vi "MOKE-4-27-22.vi"() -> ()   [LabVIEW 2021]
uses:
  <vilib>/Analysis/NI_AALBase.lvlib
  <vilib>/Analysis/baseanly.llb/Mean (DBL).vi
  <vilib>/Analysis/Matrix/Datatypes/RealMatrix.ctl
  <vilib>/Analysis/Matrix/NI_Matrix.lvlib
panel:
  out "avg":dbl
  out "y_indicator":dbl
  out "col_arr":dbl[][](array[numeric])
  in  "blank":dbl[](array[numeric])
  out "y_mat":T1
  in  "stop":bool
  in  "Total Loops":dbl
  out "Current Loop":i32
  in  "Time / Step":i64
  in  "Number of Samples":i32=100
  out "Graph For Photodiode":cluster{"Y":dbl[], "Y":dbl[]}[](graph)
  out "Photodiode Level":dbl
  out "Current Voltage":dbl
  in  "Scans From 0 to Max Voltage":i32
  in  "Voltage":dbl
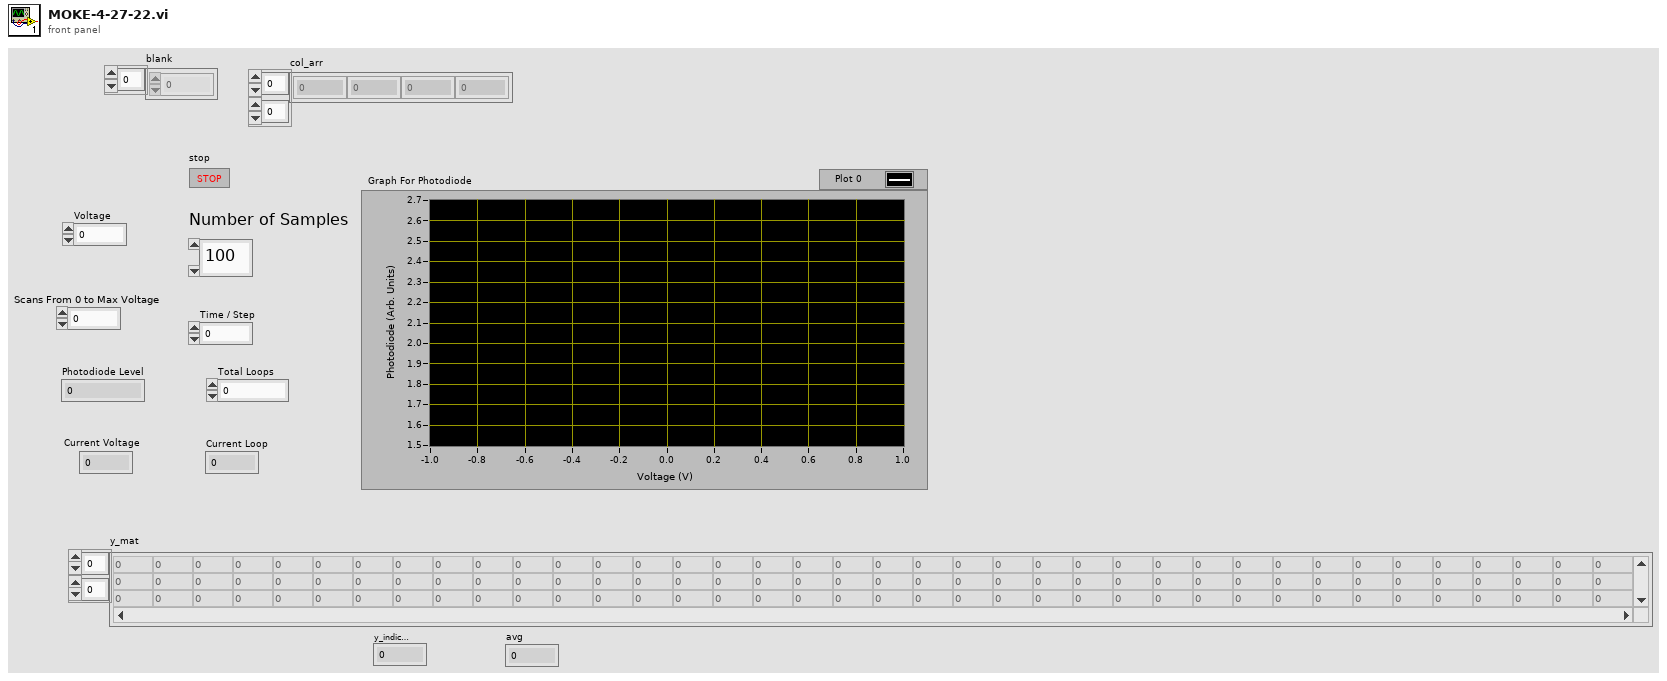
[diagram p1: front panel]
types:
  T1 = typedef "NI_Matrix.lvlib/RealMatrix.ctl" = dbl[][]
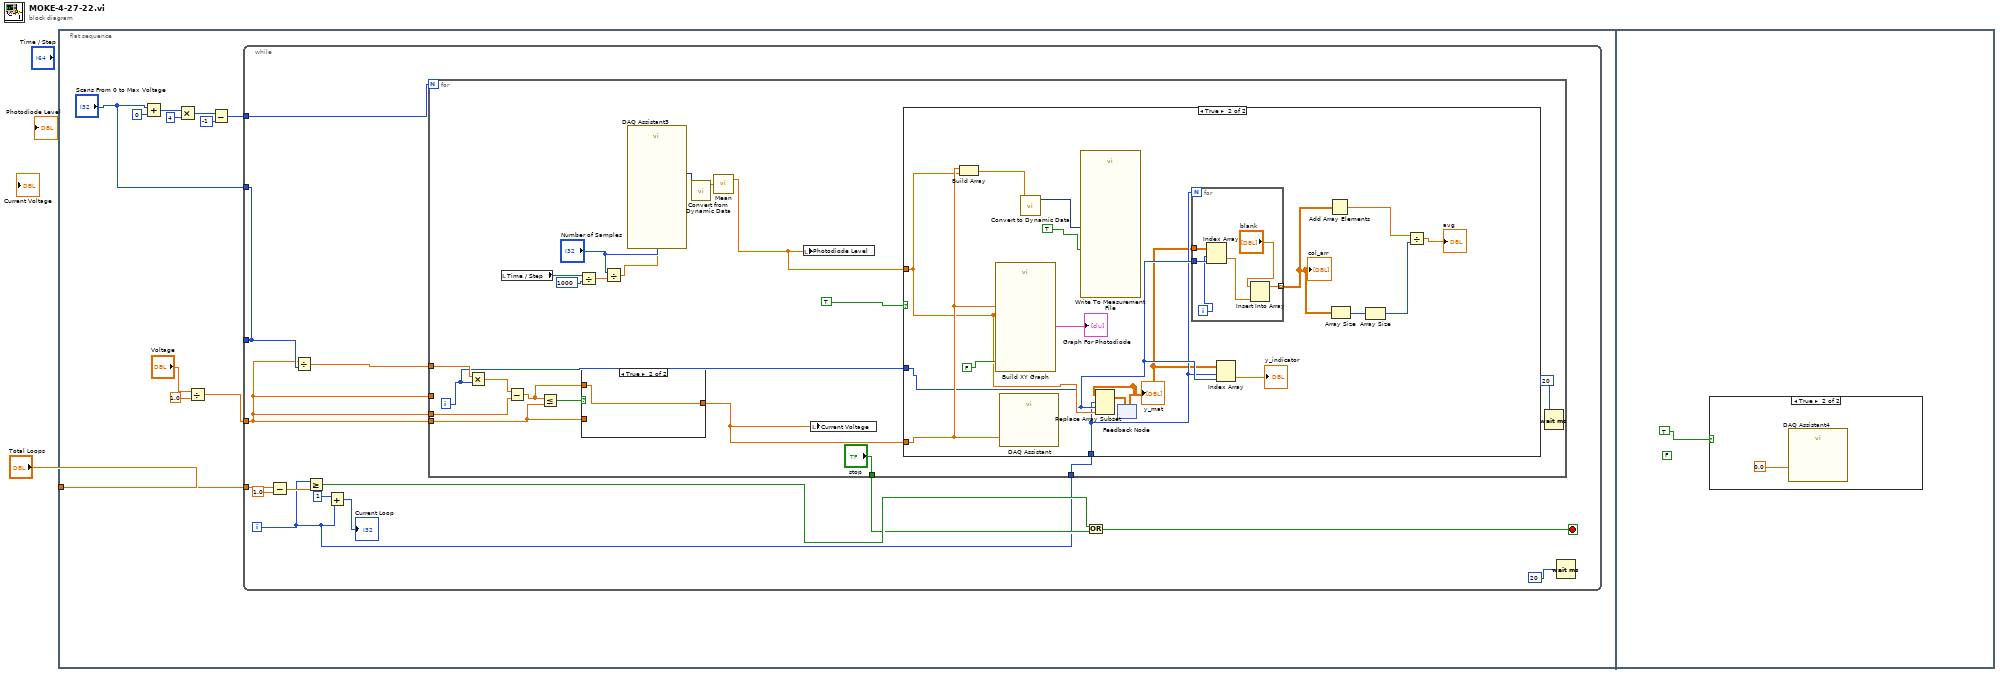
[diagram p0: block diagram]
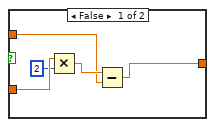
[diagram p2: hidden frame]
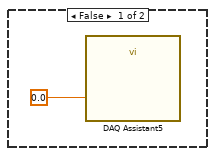
[diagram p4: hidden frame]
diagram:
  n1 = flat-sequence {
    tunnel: "Total Loops" -> [w5]
    frame #0 {
      n2 = Add(x="Scans From 0 to Max Voltage", y=0) -> (x+y=w11:i32)
      n3 = Multiply(x=w11, y=4) -> (x*y=w12:i32)
      n4 = Divide(x="Voltage", y=1.0) -> (x/y=w2:dbl)
      n5 = Subtract(x=w12, y=-1) -> (x-y=w7:i32)
      n6 = while {
        tunnel: w5 -> [w25]
        tunnel: [w16] -> _
        tunnel: w7 -> [w17]
        tunnel: "Scans From 0 to Max Voltage" -> [w16]
        tunnel: w2 -> [w15]
        i -> [w13]
        stop <- w19 stop-if-true
        n7 = Subtract(x=w25, y=1.0) -> (x-y=w24:dbl)
        n8 = Divide(x=w15, y=w16) -> (x/y=w26:dbl)
        n9 = Greater Or Equal?(x=w13, y=w24) -> (x >= y?=w20:bool)
        n10 = Add(x=1, y=w13) -> (x+y=→"Current Loop":i32)
        n11 = for {
          N: w17 -> [_]
          tunnel: w26 -> [w46]
          tunnel: w15 -> [_]
          tunnel: w15 -> [w43]
          tunnel: w15 -> [w39]
          tunnel: ["stop"] -> w18
          tunnel: w13 -> [w27]
          i -> [w28]
          n12 = Multiply(x=w46, y=w28) -> (x*y=w44:dbl)
          n13 = local read "Time / Step"() -> (w35:i64)
          n14 = Subtract(x=w44, y=w43) -> (x-y=w41:dbl)
          n15 = Less Or Equal?(x=w41, y=w39) -> (x <= y?=w42:bool)
          n16 = Divide(x=w35, y=i64 1000) -> (x/y=w36:dbl)
          n17 = case shown="True" w42 {
            tunnel: w41 -> [w48 w52]
            tunnel: [w47 w52] -> w40
            tunnel: w39 -> [w51 _]
            frame False {
              n18 = Multiply(x=w51, y=2) -> (x*y=w49:dbl)
              n19 = Subtract(x=w49, y=w48) -> (x-y=w47:dbl)
            }
            frame True {
            }
          }
          n20 = Divide(x="Number of Samples", y=w36) -> (x/y=w37:dbl)
          n21 = call "DAQ Assistant3"("rate"=w37, "number of samples"="Number of Samples") -> ("data"=w33:dynamicdata)  [unwired: 4 in, 13 out]
          n22 = call "Convert from Dynamic Data"("Dynamic Data Type"=w33) -> ("Array"=w32:dbl[])  [unwired: 3 in]
          n23 = call-poly <vilib>:"Mean.vi"("X"=w32) -> ("mean"=w31:dbl)  [unwired: 1 out]
          n24 = local write "Photodiode Level"(w31) -> ()
          n25 = local write "Current Voltage"(w40) -> ()
          n26 = case shown="True" TRUE {
            tunnel: w40 -> [_ w68]
            tunnel: w31 -> [_ w63]
            tunnel: w28 -> [_ w61]
            tunnel: w27 -> [_ w60]
            frame False {
            }
            frame True {
              n27 = Build Array(w68, w63) -> (w66:dbl[])
              n28 = call "Build XY Graph"("Reset"=FALSE, "Y Input"=w63, "X Input"=w68) -> ("XY Graph"=→"Graph For Photodiode":cluster{"X":dbl[], "Y":dbl[]}[])  [unwired: 7 in, 1 out]
              n29 = call "DAQ Assistant"("data"=w68) -> ()  [unwired: 17 in, 2 out]
              n30 = call "Convert to Dynamic Data"("Array"=w66) -> ("Dynamic Data Type"=w64:dynamicdata)  [unwired: 3 in]
              n31 = call "Write To Measurement File"("Signals"=w64, "Enable"=TRUE) -> ()  [unwired: 15 in, 3 out]
              n32 = feedback #1() -> (w59:T1)  [unwired: 1 in]
              "y_mat" <- w59
              n33 = Replace Array Subset(array=w59, new element=w63, index (row)=w60, index (col)=w61) -> (w62:T1)
              n34 = feedback-in #1(w62) -> ()
              n35 = for {
                N: w60 -> [_]
                tunnel: w59 -> [w75]
                tunnel: w61 -> [w71]
                tunnel: [w72] -> w57 mode=indexing
                i -> [w70]
                n36 = Index Array(array=w75, index (row)=w70, index (col)=w71) -> (element=w74:dbl)
                n37 = Insert Into Array(array="blank", new element=w74) -> (w72:dbl[])  [unwired: 1 in]
              }
              "col_arr" <- w57
              n38 = Index Array(array=w59, index (row)=w60, index (col)=w61) -> (element=→"y_indicator":dbl)
              n39 = Add Array Elements(numeric array=w57) -> (sum=w56:dbl)
              n40 = Array Size(array=w57) -> (size(s)=w55:i32[])
              n41 = Array Size(array=w55) -> (size(s)=w54:i32)
              n42 = Divide(x=w56, y=w54) -> (x/y=→"avg":dbl)
            }
          }
          n43 = Wait (ms)(milliseconds to wait=20) -> ()  [unwired: 1 out]
        }
        n44 = Or(x=w20, y=w18) -> (x .or. y?=w19:bool)
        n45 = Wait (ms)(milliseconds to wait=u32 20) -> ()  [unwired: 1 out]
      }
    }
    frame #1 {
      (unwired) FALSE
      n46 = case shown="True" TRUE {
        frame False {
          n47 = call "DAQ Assistant5"("data"=0.0) -> ()  [unwired: 17 in, 2 out]
        }
        frame True {
          n48 = call "DAQ Assistant4"("data"=0.0) -> ()  [unwired: 17 in, 2 out]
        }
      }
    }
  }
